vi "CheckType.vi"(10 "Class Name":string, 11 "types":T1) -> (3 "TypeMatch":bool)   [LabVIEW 2013, in "GenLVOOP.lvclass"]
uses:
  GenLVOOP.lvclass
  baseClass/types.ctl
  baseClass/baseClass.lvclass
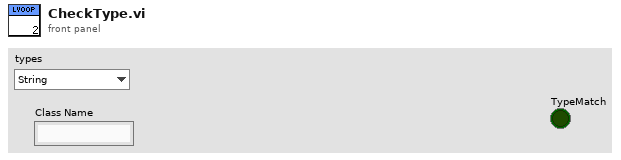
[diagram p1: front panel]
types:
  T1 = typedef "baseClass.lvclass/types.ctl" = enum16{"String", "Int32", "Uint32", "Array", "Class", "Double", "Enum"}
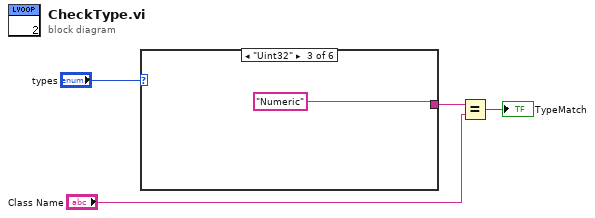
[diagram p0: block diagram]
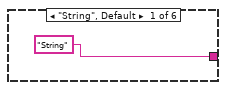
[diagram p2: hidden frame]
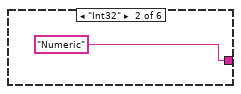
[diagram p3: hidden frame]
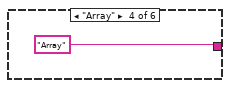
[diagram p4: hidden frame]
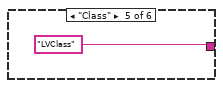
[diagram p5: hidden frame]
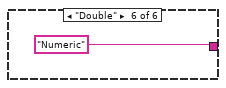
[diagram p6: hidden frame]
diagram:
  n1 = case shown="\"Uint32\"" "types" {
    tunnel: ["String" "Numeric" "Numeric" "Array" "LVClass" "Numeric"] -> w3
    frame "String", Default {
    }
    frame "Int32" {
    }
    frame "Uint32" {
    }
    frame "Array" {
    }
    frame "Class" {
    }
    frame "Double" {
    }
  }
  n2 = Equal?(x=w3, y="Class Name") -> (x = y?=→"TypeMatch":bool)
